vi "Global LM model function and gradient (2-Exp, Convolved, Periodic).vi"(3 "output control":T1, 4 "data":variant, 5 "X":dbl[](array[numeric]), 6 "a":dbl[](array[numeric])) -> (0 "error out":errorcluster, 1 "f'(X,a)":dbl[][](array[numeric]), 2 "f(X,a)":dbl[](array[numeric]))   [LabVIEW 2021, in "Fits.lvlib"]
doc: "This template is the starting point for creating a model function to be passed to the Nonlinear Curve Fit.vi."
uses:
  Fits.lvlib
  <vilib>/gmath/NumericalOptimization/LM_output select.ctl
  Global Fits/Global Fit Data.ctl
  Global Fits/Global Fit Parameters Information.ctl
  <vilib>/gmath/NI_Gmath.lvlib
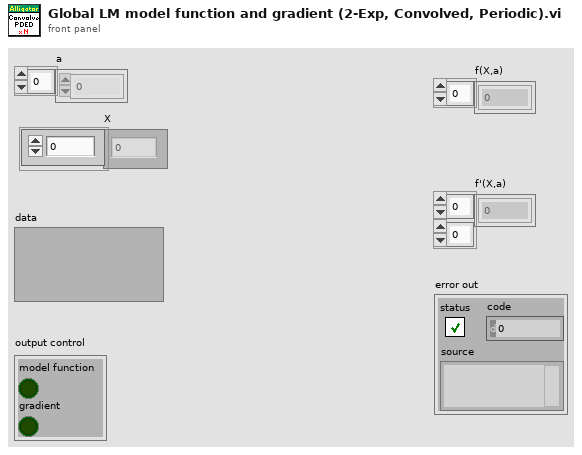
[diagram p1: front panel]
types:
  T1 = typedef "NI_Gmath.lvlib/LM_output select.ctl" = cluster{"model function":bool, "gradient":bool}
  T2 = typedef "Fits.lvlib/Global Fit Data.ctl" = cluster{"Fit Data":variant, "Global Fit Parameter Information":T3, "# Points in Plots":i32[]}
  T3 = typedef "Fits.lvlib/Global Fit Parameters Information.ctl" = cluster{"Original Parameter Indices":i32[], "# Global Parameters":i32, "# Plot Specific Parameters":i32, "Global Parameter? Array":bool[]}
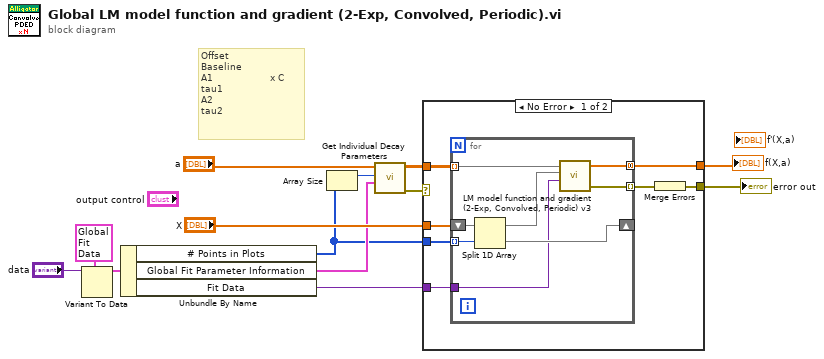
[diagram p0: block diagram]
diagram:
  # "Offset \nBaseline\nA1                   x C\ntau1\nA2\ntau2"
  n1 = Variant To Data(type=T2 {"Fit Data"=variant(cluster{"t Array":dbl[], "IRF Array":dbl[]} {"t Array"=[], "IRF Array"=[]}), "Global Fit Parameter Information"={"Original Parameter Indices"=[], "# Global Parameters"=0, "# Plot Specific Parameters"=0, "Global Parameter? Array"=[]}, "# Points in Plots"=[]} ("IRF"), Variant="data") -> (data=w10:T2)  [unwired: 1 in, 1 out]
  n2 = Unbundle By Name(w10) -> ("# Points in Plots"=w7:i32[], "Global Fit Parameter Information"=w8:T3, "Fit Data"=w3:variant)
  n3 = Array Size(array=w7) -> (size(s)=w5:i32)
  n4 = call "Get Individual Decay Parameters.vi"("Global Fit Parameter Info"=w8, "# Decays"=w5, "Global Fit Parameters Array"="a") -> ("Error Out"=w4:errorcluster, "All Parameters Array"=w6:dbl[][])  [unwired: 5 in, 2 out]
  n5 = case shown="No Error" w4 {
    selector: w4 -> [_ w29]
    tunnel: "X" -> [w20 _]
    tunnel: w7 -> [w19 _]
    tunnel: w6 -> [w18 _]
    tunnel: w3 -> [w17 _]
    tunnel: [w16 _] -> w2
    tunnel: [w14 w29] -> w1
    frame No Error {
      n6 = for {
        tunnel: w18 -> [w25] mode=indexing
        shift-right: [w26] -> _
        shift-left: w20 -> [w28]
        tunnel: w19 -> [w27] mode=indexing
        tunnel: w17 -> [w23]
        tunnel: [w22] -> w16 mode=concatenating
        tunnel: [w21] -> w15 mode=indexing
        n7 = Split 1D Array(array=w28, index=w27) -> (first subarray=w24:dbl[], second subarray=w26:dbl[])
        n8 = call "LM model function and gradient (2-Exp, Convolved, Periodic) v3.vi"("data"=w23, "X"=w24, "a"=w25) -> ("error out"=w21:errorcluster, "f(X,a)"=w22:dbl[])  [unwired: 1 in, 1 out]
      }
      n9 = Merge Errors(w15) -> (w14:errorcluster)
    }
    frame Error {
    }
  }
  "f(X,a)" <- w2
  "error out" <- w1
